vi "Generate parameters.vi"(0 "Wavenet-IIR Parameters":T4={"Activation function, fn"=0, "Neurons, J"=1, "Feedbacks, Q"=1, "Feedforwards, R"=1, "Inputs, I"=1, "Outputs, P"=1, "Weights, hW"=0.0, "Feedbacks, ha"=0.0, "Forwards, hb"=0.0, "Scalings, hA"=0.0, "Shiftings, hB"=0.0, "Persistan signal, ps"=0.0} {"Persistan signal, ps" format="%.2e"; "Shiftings, hB" format="%.2e"; "Scalings, hA" format="%.2e"; "Forwards, hb" format="%.2e"; "Feedbacks, ha" format="%.2e"; "Weights, hW" format="%.2e"; "Outputs, P" min=1 max=10 step=1; "Inputs, I" min=1 max=10 step=1; "Feedforwards, R" min=1 max=10 step=1; "Feedbacks, Q" min=1 max=10 step=1; "Neurons, J" min=1 max=10 step=1; "Activation function, fn" items=["Morlet", "RASP1", "RASP2", "RASP3", "POLYWOG1", "POLYWOG2", "POLYWOG3", "POLYWOG4", "POLYWOG5", "Shannon", "Atomic", "Flat top 1", "Flat top 2", "Flat top 3", "Flat top 4", "Flat top 5", "Flat top 6", "Hanning", "Hamming", "Blackman", "Blackman-Harris"]}, 1 "Samples, re":i32=1 min=1 max=100 step=1) -> (2 "Wavenet-IIR Behavior":T3 {"Function, dy" format="%.3f"; "Function, y" format="%.3f"; "Tau, t" format="%.3f"; "Forwards, D" format="%.3f"; "Feedbacks, C" format="%.3f"; "Weights, W" format="%.3f"; "Shifts, B" format="%.3f"; "Scales, A" format="%.3f"}, 3 "Wavenet-IIR Gradients":T2 {"Forwards, D" format="%.3f"; "Feedbacks, C" format="%.3f"; "Weights, W" format="%.3f"; "Shifts, B" format="%.3f"; "Scales, A" format="%.3f"}, 4 "Wavenet-IIR Memories":T1 {"Activation functions, dF" format="%.3f"; "Wavenet, Z" format="%.3f"; "Tracking errors, e" format="%.3f"; "Activation functions, F" format="%.3f"; "Wavenet-IIR, Y" format="%.3f"})   [LabVIEW 2022 SP3]
panel:
  out "Tau, t":dbl[](array[numeric]) format="%.3f"
  out "Forwards, D":dbl[][](array[numeric]) format="%.3f"
  out "Feedbacks, C":dbl[][](array[numeric]) format="%.3f"
  out "Weights, W":dbl[][](array[numeric]) format="%.3f"
  out "Shifts, B":dbl[](array[numeric]) format="%.3f"
  out "Scales, A":dbl[](array[numeric]) format="%.3f"
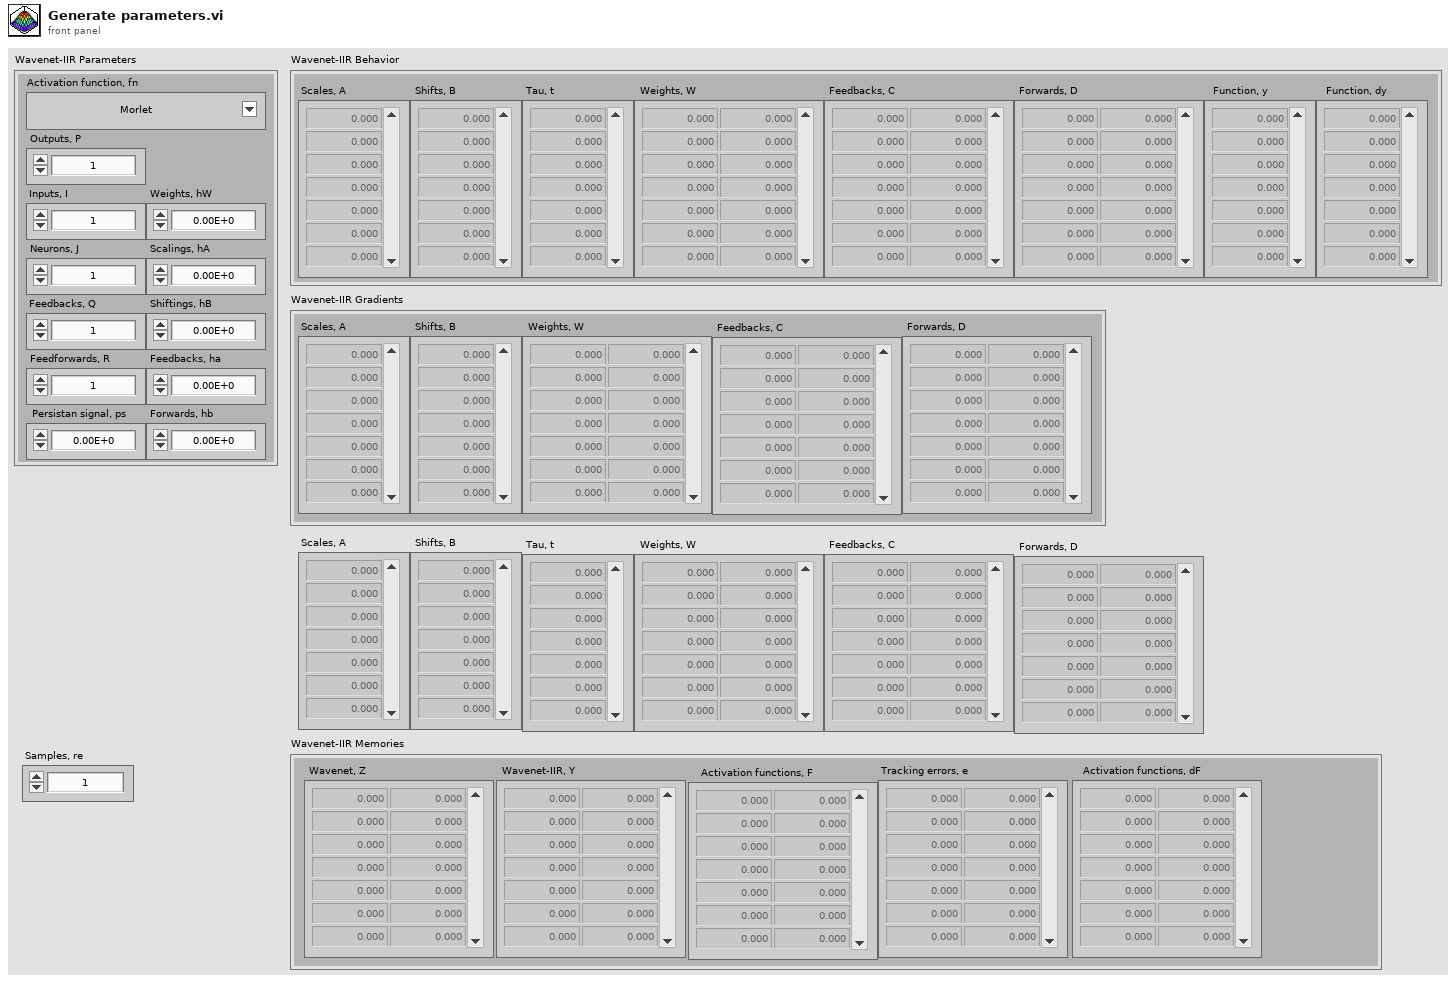
[diagram p1: front panel]
types:
  T1 = cluster{"Wavenet-IIR, Y":dbl[][], "Activation functions, F":dbl[][], "Tracking errors, e":dbl[][], "Wavenet, Z":dbl[][], "Activation functions, dF":dbl[][]}
  T2 = cluster{"Scales, A":dbl[], "Shifts, B":dbl[], "Weights, W":dbl[][], "Feedbacks, C":dbl[][], "Forwards, D":dbl[][]}
  T3 = cluster{"Scales, A":dbl[], "Shifts, B":dbl[], "Weights, W":dbl[][], "Feedbacks, C":dbl[][], "Forwards, D":dbl[][], "Tau, t":dbl[], "Function, y":dbl[], "Function, dy":dbl[]}
  T4 = cluster{"Activation function, fn":u16, "Neurons, J":i32, "Feedbacks, Q":i32, "Feedforwards, R":i32, "Inputs, I":i32, "Outputs, P":i32, "Weights, hW":dbl, "Feedbacks, ha":dbl, "Forwards, hb":dbl, "Scalings, hA":dbl, "Shiftings, hB":dbl, "Persistan signal, ps":dbl}
  T5 = typedef "NI_Matrix.lvlib/RealMatrix.ctl" = dbl[][]
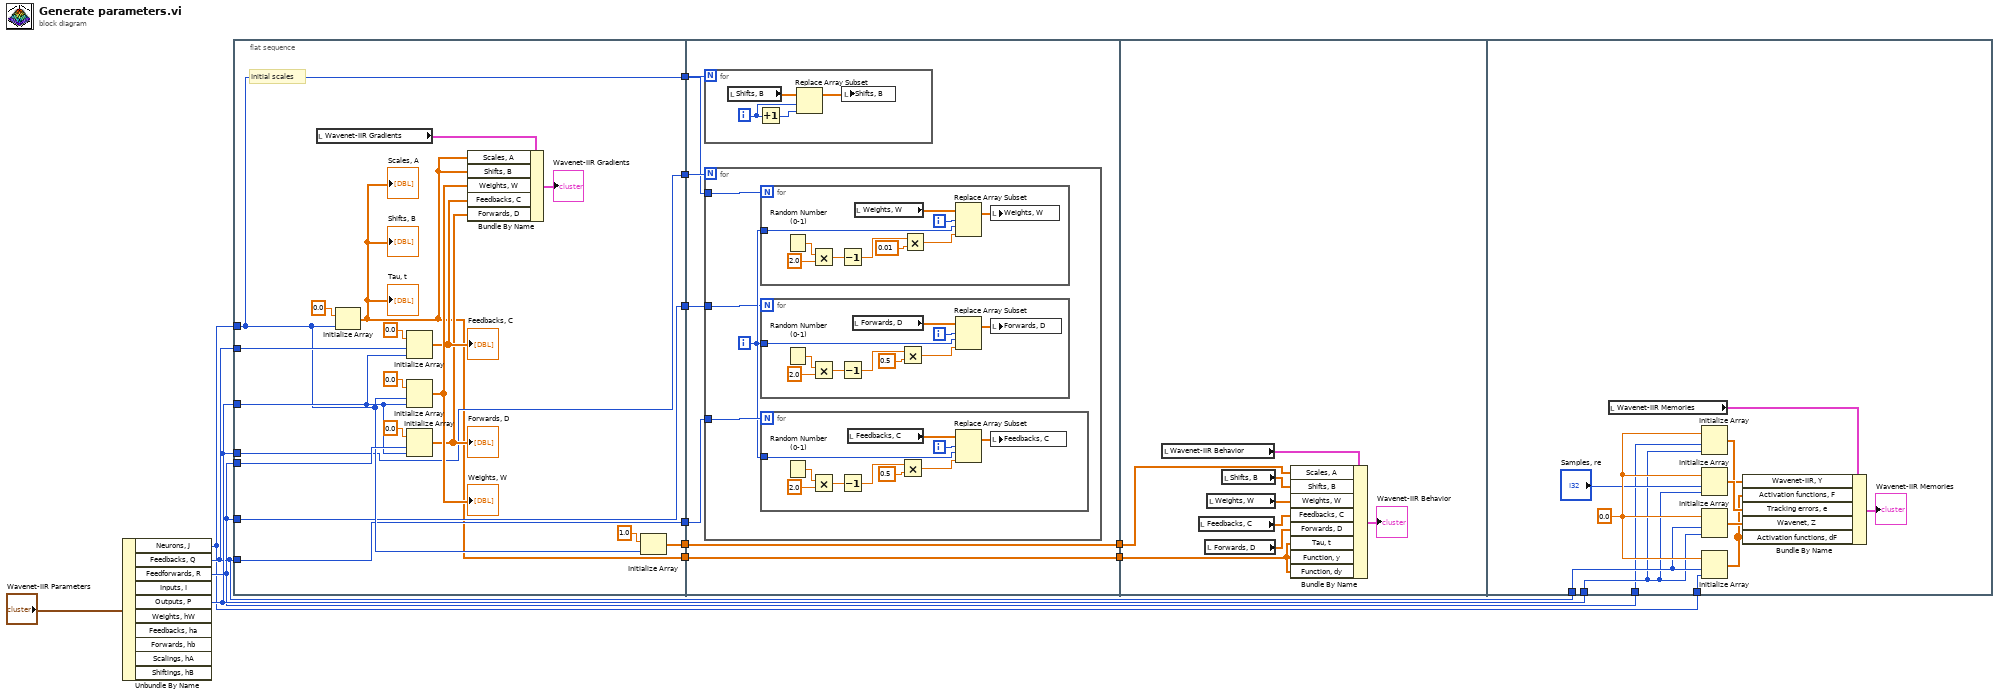
[diagram p0: block diagram]
diagram:
  n1 = Unbundle By Name("Wavenet-IIR Parameters") -> ("Neurons, J"=w1:i32, "Feedbacks, Q"=w2:i32, "Feedforwards, R"=w3:i32, "Outputs, P"=w4:i32)  [unwired: 6 out]
  n2 = flat-sequence {
    tunnel: w1 -> [w22]
    tunnel: w4 -> [w25]
    tunnel: w2 -> [w28]
    tunnel: w3 -> [w26]
    tunnel: [w22] -> w12
    tunnel: [w18] -> w10
    tunnel: [w14] -> w8
    tunnel: w4 -> [w17]
    tunnel: [w17] -> w7
    tunnel: w2 -> [w16]
    tunnel: [w16] -> w6
    tunnel: w3 -> [w15]
    tunnel: [w15] -> w5
    tunnel: w12 -> [w35]
    tunnel: [w38] -> w11
    tunnel: w10 -> [w38]
    tunnel: [w37] -> w9
    tunnel: w8 -> [w37]
    tunnel: w7 -> [w36]
    tunnel: w6 -> [w34]
    tunnel: w5 -> [w33]
    tunnel: w11 -> [w78]
    tunnel: w9 -> [w77]
    tunnel: w4 -> [w87]
    tunnel: w2 -> [w90]
    tunnel: w3 -> [w86]
    tunnel: w1 -> [w89]
    frame #0 {
      # "Initial scales"
      n3 = local read "Wavenet-IIR Gradients"() -> (w23:T2)
      n4 = Initialize Array(0.0 ("element"), w22) -> (w14:dbl[])
      "Scales, A" <- w14
      "Shifts, B" <- w14
      "Tau, t" <- w14
      n5 = Initialize Array(0.0 ("element"), w28, w25) -> (w20:dbl[][])
      "Feedbacks, C" <- w20
      n6 = Initialize Array(0.0 ("element"), w22, w25) -> (w21:dbl[][])
      "Weights, W" <- w21
      n7 = Initialize Array(0.0 ("element"), w26, w25) -> (w19:dbl[][])
      "Forwards, D" <- w19
      n8 = Bundle By Name(cluster=w23, "Scales, A"=w14, "Shifts, B"=w14, "Weights, W"=w21, "Feedbacks, C"=w20, "Forwards, D"=w19) -> (→"Wavenet-IIR Gradients":T2)
      n9 = Initialize Array(1.0 ("element"), w22) -> (w18:dbl[])
    }
    frame #1 {
      n10 = for {
        N: w35 -> [_]
        i -> [w74]
        n11 = local read "Shifts, B"() -> (w76:dbl[])
        n12 = Increment(x=w74) -> (x+1=w75:i32)
        n13 = Replace Array Subset(array=w76, new element=w75, index=w74) -> (w73:dbl[])
        n14 = local write "Shifts, B"(w73) -> ()
      }
      n15 = for {
        N: w36 -> [_]
        tunnel: w35 -> [w42]
        tunnel: w34 -> [w41]
        tunnel: w33 -> [w39]
        i -> [w40]
        n16 = for {
          N: w42 -> [_]
          tunnel: w40 -> [w63]
          i -> [w64]
          n17 = Random Number (0-1)() -> (number: 0 to 1=w68:dbl)
          n18 = Multiply(x=w68, y=2.0) -> (x*y=w67:dbl)
          n19 = Decrement(x=w67) -> (x-1=w66:dbl)
          n20 = local read "Weights, W"() -> (w72:dbl[][])
          n21 = Multiply(x=w66, y=0.01) -> (x*y=w65:dbl)
          n22 = Replace Array Subset(array=w72, new element=w65, index (row)=w64, index (col)=w63) -> (w71:T5)
          n23 = local write "Weights, W"(w71) -> ()
        }
        n24 = for {
          N: w39 -> [_]
          tunnel: w40 -> [w43]
          i -> [w44]
          n25 = Random Number (0-1)() -> (number: 0 to 1=w50:dbl)
          n26 = Multiply(x=w50, y=2.0) -> (x*y=w52:dbl)
          n27 = Decrement(x=w52) -> (x-1=w51:dbl)
          n28 = local read "Forwards, D"() -> (w46:dbl[][])
          n29 = Multiply(x=w51, y=0.5) -> (x*y=w47:dbl)
          n30 = Replace Array Subset(array=w46, new element=w47, index (row)=w44, index (col)=w43) -> (w45:T5)
          n31 = local write "Forwards, D"(w45) -> ()
        }
        n32 = for {
          N: w41 -> [_]
          tunnel: w40 -> [w53]
          i -> [w54]
          n33 = Random Number (0-1)() -> (number: 0 to 1=w60:dbl)
          n34 = Multiply(x=w60, y=2.0) -> (x*y=w58:dbl)
          n35 = Decrement(x=w58) -> (x-1=w59:dbl)
          n36 = local read "Feedbacks, C"() -> (w56:dbl[][])
          n37 = Multiply(x=w59, y=0.5) -> (x*y=w57:dbl)
          n38 = Replace Array Subset(array=w56, new element=w57, index (row)=w54, index (col)=w53) -> (w55:T5)
          n39 = local write "Feedbacks, C"(w55) -> ()
        }
      }
    }
    frame #2 {
      n40 = local read "Wavenet-IIR Behavior"() -> (w83:T3)
      n41 = local read "Feedbacks, C"() -> (w80:dbl[][])
      n42 = local read "Forwards, D"() -> (w79:dbl[][])
      n43 = local read "Weights, W"() -> (w81:dbl[][])
      n44 = local read "Shifts, B"() -> (w82:dbl[])
      n45 = Bundle By Name(cluster=w83, "Scales, A"=w78, "Shifts, B"=w82, "Weights, W"=w81, "Feedbacks, C"=w80, "Forwards, D"=w79, "Tau, t"=w77, "Function, y"=w77, "Function, dy"=w77) -> (→"Wavenet-IIR Behavior":T3)
    }
    frame #3 {
      w94 = 0.0 ("element")
      n46 = local read "Wavenet-IIR Memories"() -> (w96:T1)
      n47 = Initialize Array(w94, w86, w87) -> (w88:dbl[][])
      n48 = Initialize Array(w94, "Samples, re", w87) -> (w92:dbl[][])
      n49 = Initialize Array(w94, w90, w87) -> (w91:dbl[][])
      n50 = Initialize Array(w94, w90, w89) -> (w85:dbl[][])
      n51 = Bundle By Name(cluster=w96, "Wavenet-IIR, Y"=w88, "Activation functions, F"=w85, "Tracking errors, e"=w92, "Wavenet, Z"=w91, "Activation functions, dF"=w85) -> (→"Wavenet-IIR Memories":T1)
    }
  }
